vi "get steady state voltage - diode.vi"(9 "Reignition Task In":refnum<k21>, 10 "Diode Task In":refnum<k21>, 11 "RF Generator Task In":refnum<k21>) -> (0 "Output":dbl, 1 "reignition task out":refnum<k21>, 2 "diode task out":refnum<k21>, 3 "rf generator task out":refnum<k21>)   [LabVIEW 2018]
uses:
  <vilib>/DAQmx/write.llb/DAQmx Write (Analog DBL 1Chan 1Samp).vi
  0537a0e4-9a25-4750-8707-345dd33cb303.vi
  2318391d-fd01-44f5-9c85-a6517690b298.vi
  <vilib>/DAQmx/read.llb/DAQmx Read (Analog DBL 1Chan 1Samp).vi
  <vilib>/DAQmx/miscellaneous.llb/DAQmx Fill In Error Info.vi
  <vilib>/Analysis/NI_AALBase.lvlib
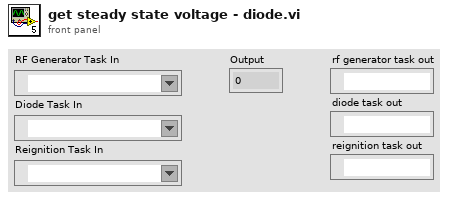
[diagram p1: front panel]
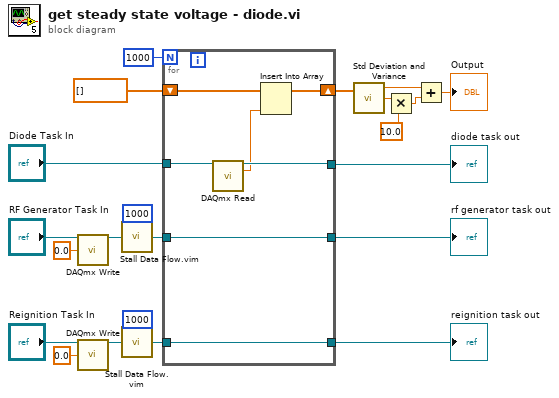
[diagram p0: block diagram]
diagram:
  n1 = call-poly <vilib>:"DAQmx Write.vi"("task/channels in"="RF Generator Task In", "data"=0.0) -> ("task out"=w13:refnum<k21>)  [unwired: 11 in, 2 out]
  n2 = call-poly <vilib>:"DAQmx Write.vi"("task/channels in"="Reignition Task In", "data"=0.0) -> ("task out"=w6:refnum<k21>)  [unwired: 11 in, 2 out]
  n3 = call "Stall Data Flow.vim"("value in"=w13, "milliseconds to wait"=u32 1000) -> ("value out"=w8:refnum<k21>)  [unwired: 1 out]
  n4 = call "Stall Data Flow.vim"("value in"=w6, "milliseconds to wait"=u32 1000) -> ("value out"=w2:refnum<k21>)  [unwired: 1 out]
  n5 = for {
    N: 1000 -> [_]
    shift-right: [w25] -> w20
    shift-left: dbl[] [] ("Y") -> [w27]
    tunnel: [w29] -> w18
    tunnel: [w28] -> w14
    tunnel: w8 -> [w28]
    tunnel: "Diode Task In" -> [w24]
    tunnel: w2 -> [w23]
    tunnel: [w23] -> w1
    n6 = call-poly <vilib>:"DAQmx Read.vi"("task/channels in"=w24) -> ("task out"=w29:refnum<k21>, "data"=w26:dbl)  [unwired: 12 in, 1 out]
    n7 = Insert Into Array(array=w27, new element=w26) -> (w25:dbl[])  [unwired: 1 in]
  }
  "diode task out" <- w18
  "rf generator task out" <- w14
  "reignition task out" <- w1
  n8 = call <vilib>:"Std Deviation and Variance.vi"("X"=w20) -> ("mean"=w17:dbl, "standard deviation"=w22:dbl)  [unwired: 1 in, 1 out]
  n9 = Multiply(x=w22, y=10.0) -> (x*y=w16:dbl)
  n10 = Add(x=w17, y=w16) -> (x+y=→"Output":dbl)
